vi "Test RD Retrieval - Target - Nick.vi"() -> ()   [LabVIEW 2015]
uses:
  <vilib>/rvi/interface/nirviOpenFPGA/nirviOpenFPGA.xnode
  <vilib>/rvi/interface/nirviCloseFPGA/nirviCloseFPGA.xnode
  <vilib>/rvi/interface/nirviMethod/nirviMethod.xnode
  <vilib>/rvi/errors/niLvFpgaMergeErrorWithErrorCode.vi
  <vilib>/rvi/interface/nirviReadWriteControl/nirviReadWriteControl.xnode
  NiFpgaLv.dll
  <vilib>/Utility/error.llb/Error Cluster From Error Code.vi
  <vilib>/rvi/errors/niLvFpgaAdjustHostInterfaceError.vi
  FPGA Bitfiles/Nicholas.lvbitx
  <vilib>/FPGAPlugInAG/cRIO-9081/niLvFpga_Open_cRIO-9081.vi
  <vilib>/FPGAPlugInAG/cRIO-9081/niLvFpga_ConfigureFifo_cRIO-9081.vi
  <vilib>/FPGAPlugInAG/cRIO-9081/niLvFpga_StartFifo_cRIO-9081.vi
  <vilib>/rvi/interface/nirviMethod/StockFPGA_InlinedMethodWaitForSingleIRQ.vi
  <vilib>/FPGAPlugInAG/cRIO-9081/niLvFpga_WaitOnIrq_cRIO-9081.vi
  <vilib>/FPGAPlugInAG/cRIO-9081/niLvFpga_AcknowledgeIrq_cRIO-9081.vi
  <vilib>/FPGAPlugInAG/cRIO-9081/niLvFpga_ReadFifo_cRIO-9081.vi
  <vilib>/FPGAPlugInAG/cRIO-9081/niLvFpga_Close_cRIO-9081.vi
panel:
  out "Waveform Graph 3":sgl[](graph)
  in  "Num2Acq":u16=500
  out "Waveform Graph 2":sgl[][](graph)
  out "Waveform Chart":cluster{i32, sgl}(graph)
  in  "TotNumSamp":u16=1000
  in  "DC":u16=500
  out "error out 2":errorcluster
  out "error out":errorcluster
  out "x-y":dbl=2.071805000305176
  out "channel 0":sgl[](array[numeric])
  in  "Stop":bool
  out "Elements Remaining":u32=2903286
  in  "Number of Elements":u32=999870
  out "Actual Depth":u32=5000000
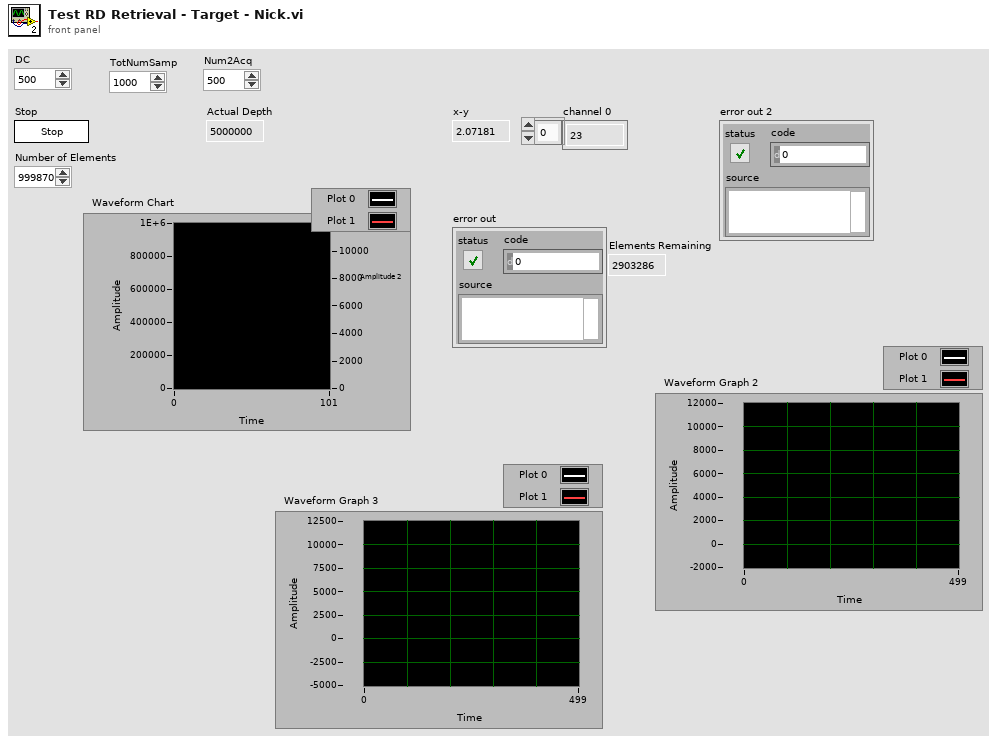
[diagram p1: front panel]
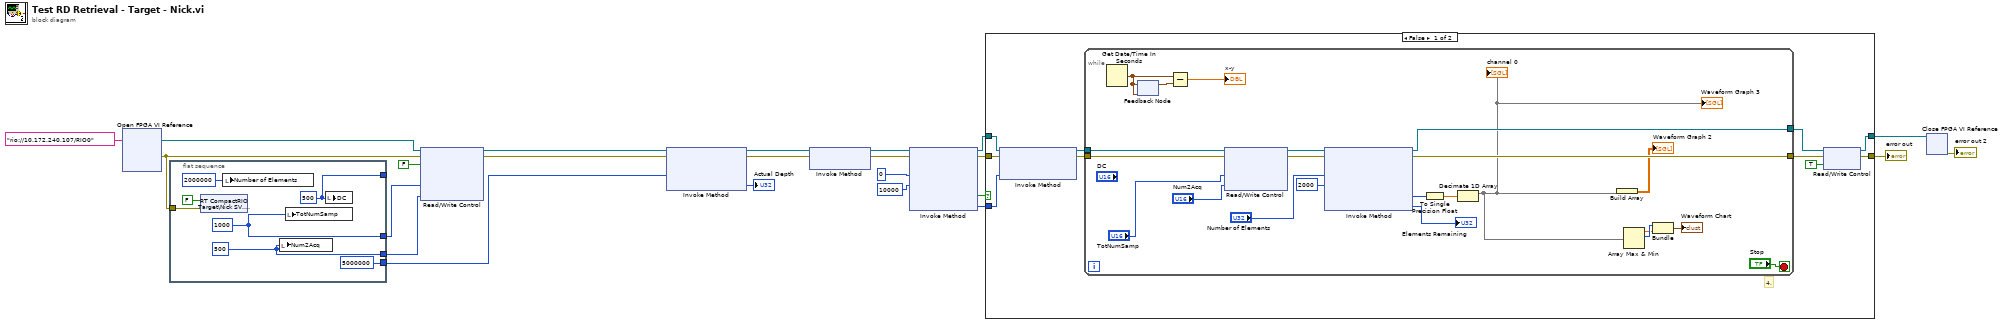
[diagram p0: block diagram]
diagram:
  n1 = xnode "Open FPGA VI Reference"("resource name"=tag "rio://10.172.240.107/RIO0") -> ("FPGA VI Reference Out"=w14:refnum<k20>, "error out"=w12:errorcluster)  [unwired: 1 in]
  n2 = flat-sequence {
    tunnel: w12 -> [w29]
    tunnel: [w28] -> w1
    tunnel: [w27] -> _
    tunnel: [u32 5000000 ("Requested Depth")] -> w5
    tunnel: [w25] -> w2
    frame #0 {
      w25 = u16 500 ("Num2Acq")
      w28 = u16 1000 ("TotNumSamp")
      w27 = u16 500 ("DC")
      n3 = shared-variable "RT CompactRIO Target\\Nick SV.lvlib\\Stop"(FALSE ("Stop"), error in=w29) -> ()  [unwired: 1 out]
      n4 = local write "Number of Elements"(u32 2000000 ("Number of Elements")) -> ()
      n5 = local write "Num2Acq"(w25) -> ()
      n6 = local write "TotNumSamp"(w28) -> ()
      n7 = local write "DC"(w27) -> ()
    }
  }
  n8 = xnode "Read/Write Control"("FPGA VI Reference In"=w14, "error in"=w12, "Stop"=FALSE, "NumSamples"=w1, "Samp2Collect"=w2) -> ("FPGA VI Reference Out"=w4:refnum<k20>, "error out"=w3:errorcluster)  [unwired: 1 in]
  n9 = xnode "Invoke Method"("FPGA VI Reference In"=w4, "error in"=w3, "Requested Depth"=w5) -> ("FPGA VI Reference Out"=w7:refnum<k20>, "error out"=w6:errorcluster, "Actual Depth"=→"Actual Depth":u32)
  n10 = xnode "Invoke Method"("FPGA VI Reference In"=w7, "error in"=w6) -> ("FPGA VI Reference Out"=w15:refnum<k20>, "error out"=w13:errorcluster)
  n11 = xnode "Invoke Method"("FPGA VI Reference In"=w15, "error in"=w13, "IRQ Number(s)"=0, "Timeout (ms)"=10000) -> ("FPGA VI Reference Out"=w21:refnum<k20>, "error out"=w22:errorcluster, "Timed Out"=w10:bool, "IRQ(s) Asserted"=w20:i32)
  n12 = case shown="False" w10 {
    tunnel: w22 -> [w40 w64]
    tunnel: w21 -> [w39 w63]
    tunnel: w20 -> [w38 _]
    tunnel: [w35 w63] -> w17
    tunnel: [w31 w64] -> w9
    frame False {
      # "4."
      n13 = xnode "Invoke Method"("FPGA VI Reference In"=w39, "error in"=w40, "IRQ Number(s)"=w38) -> ("FPGA VI Reference Out"=w37:refnum<k20>, "error out"=w33:errorcluster)
      n14 = while {
        tunnel: w37 -> [w52]
        tunnel: [w49] -> w36
        tunnel: w33 -> [w51]
        tunnel: [w48] -> w32
        stop <- "Stop" stop-if-true
        n15 = Get Date/Time In Seconds() -> (seconds since 1Jan1904=w59:timestamp)
        n16 = feedback-in #1(w59) -> ()
        n17 = feedback #1(w59) -> (w62:timestamp)
        n18 = Subtract(x=w59, y=w62) -> (x-y=→"x-y":dbl)
        n19 = xnode "Read/Write Control"("FPGA VI Reference In"=w52, "error in"=w51, "NumSamples"="TotNumSamp", "Samp2Collect"="Num2Acq") -> ("FPGA VI Reference Out"=w45:refnum<k20>, "error out"=w50:errorcluster)  [unwired: 1 in]
        n20 = xnode "Invoke Method"("FPGA VI Reference In"=w45, "error in"=w50, "Number of Elements"="Number of Elements", "Timeout (ms)"=2000) -> ("FPGA VI Reference Out"=w49:refnum<k20>, "error out"=w48:errorcluster, "Data"=w58:i16[], "Elements Remaining"=→"Elements Remaining":u32)
        n21 = To Single Precision Float(number=w58) -> (single precision float=w60:sgl[])
        n22 = Decimate 1D Array(w60) -> (w41:sgl[])  [unwired: 1 out]
        "channel 0" <- w41
        "Waveform Graph 3" <- w41
        n23 = Build Array(w41) -> (→"Waveform Graph 2":sgl[][])
        n24 = Array Max & Min(array=w41) -> (max value=w54:sgl, max index (indices)=w55:i32)  [unwired: 2 out]
        n25 = Bundle(w55, w54) -> (→"Waveform Chart":cluster{i32, sgl})  [unwired: 1 in]
      }
      n26 = xnode "Read/Write Control"("FPGA VI Reference In"=w36, "error in"=w32, "Stop"=TRUE) -> ("FPGA VI Reference Out"=w35:refnum<k20>, "error out"=w31:errorcluster)
    }
    frame True {
    }
  }
  "error out" <- w9
  n27 = xnode "Close FPGA VI Reference"("FPGA VI Reference In"=w17) -> ("error out"=→"error out 2":errorcluster)  [unwired: 1 in]
